vi "Get All Project VI Data.vi"(8 "error in":errorcluster, 11 "Lvproj Path":path) -> (0 "error out":errorcluster, 3 "VI Data":T1[](array[typedef]))   [LabVIEW 2020, in "VI Properties Editor.lvlib"]
doc: "Gets all VI data from a project located at <B>Path</B>."
uses:
  VI Properties Editor.lvlib
  <vilib>/xml/NI_XML.lvlib
  <vilib>/xml/Close Reference(Node).vi
  CTLs/Control Properties.ctl
  <vilib>/picture/picture.llb/imagedata.ctl
  CTLs/VI Properties.ctl
  CTLs/VI Data.ctl
  CTLs/XPath Get Attribute.ctl
  <vilib>/xml/Load XML String.vi
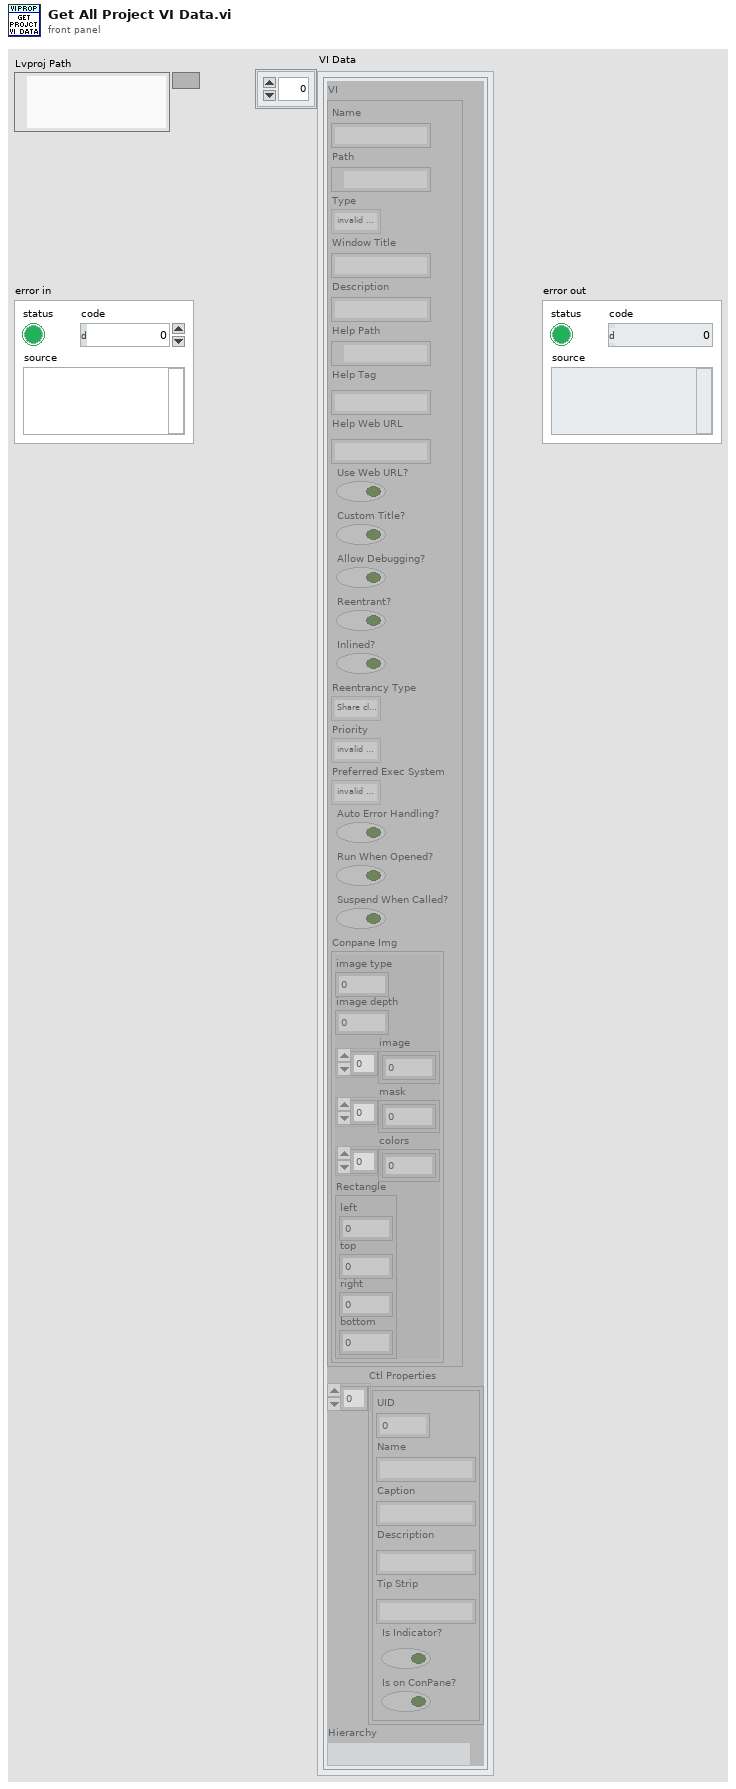
[diagram p1: front panel]
types:
  T1 = typedef "VI Properties Editor.lvlib/VI Data.ctl" = cluster{"VI":T2, "Ctl Properties":T4[], "Hierarchy":string}
  T2 = typedef "VI Properties Editor.lvlib/VI Properties.ctl" = cluster{"Name":string, "Path":path, "Type":enum32{"invalid VI type", "Standard VI", "Control VI", "Global VI", "Polymorphic VI", "Configuration VI", "SubSystem", "Facade VI", "Method VI", "Statechart Diagram VI"}, "Window Title":string, "Description":string, "Help Path":path, "Help Tag":string, "Help Web URL":string, "Use Web URL?":bool, "Custom Title?":bool, "Allow Debugging?":bool, "Reentrant?":bool, "Inlined?":bool, "Reentrancy Type":enum16{"Share clones between instances", "Preallocate clone for each instance"}, "Priority":enum32{"invalid priority", "background priority", "normal priority", "above normal priority", "high priority", "time critical priority", "subroutine"}, "Preferred Exec System":enum32{"invalid execution system", "user interface", "standard", "instrument i/o", "data acquisition", "other 1", "other 2", "same as caller"}, "Auto Error Handling?":bool, "Run When Opened?":bool, "Suspend When Called?":bool, "Conpane Img":T3}
  T3 = typedef "imagedata.ctl" = cluster{"image type":i32, "image depth":i32, "image":u8[], "mask":u8[], "colors":u32[], "Rectangle":cluster{"left":i16, "top":i16, "right":i16, "bottom":i16}}
  T4 = typedef "VI Properties Editor.lvlib/Control Properties.ctl" = cluster{"UID":i32, "Name":string, "Caption":string, "Description":string, "Tip Strip":string, "Is Indicator?":bool, "Is on ConPane?":bool}
  T5 = typedef "VI Properties Editor.lvlib/XPath Get Attribute.ctl" = enum16{"Item[@Type='VI']/@URL", "Item[@Type='LVClass']/@URL", "Item[@Type='Library']/@URL", "Item[@Type='Folder' and not (@URL)]/@Name", "@Name"}
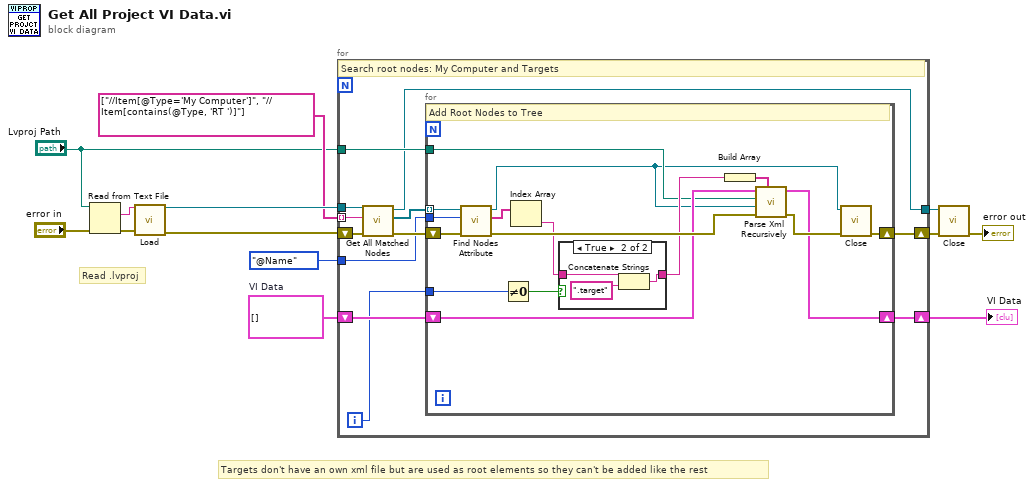
[diagram p0: block diagram]
diagram:
  w2 = T1[] []  # VI Data
  # "Targets don't have an own xml file but are used as root elements so they can't be added like the rest"
  # "Read .lvproj"
  n1 = Read from Text File(file (use dialog)="Lvproj Path", error in="error in") -> (text=w12:string, error out=w11:errorcluster)  [unwired: 2 in, 2 out]
  n2 = call-poly <vilib>:"Load.vi"("XML string"=w12, "error in (no error)"=w11) -> ("DOM document out"=w13:refnum<k20>, "error out"=w9:errorcluster)  [unwired: 11 in, 1 out]
  n3 = for {
    tunnel: w13 -> [w25]
    tunnel: string[] ["//Item[@Type='My Computer']", "//Item[contains(@Type, 'RT ')]"] -> [w24] mode=indexing
    tunnel: "Lvproj Path" -> [w23]
    shift-right: [w22] -> w10
    shift-left: w9 -> [w20]
    tunnel: [w18] -> w7
    shift-right: [w16] -> w1
    shift-left: w2 -> [w17]
    tunnel: XPath_Get_Attribute."@Name" ("XPath") -> [w15]
    i -> [w14]
    # "Search root nodes: My Computer and Targets"
    n4 = call <vilib>:"Get All Matched Nodes.vi"("error in (no error)"=w20, "XPath expression"=w24, "node in"=w25) -> ("error out"=w19:errorcluster, "node result array"=w21:refnum<k20>[], "node out"=w18:refnum<k20>)  [unwired: 6 in]
    n5 = for {
      tunnel: w23 -> [w29]
      tunnel: w21 -> [w28] mode=indexing
      shift-right: [w40] -> w22
      shift-left: w19 -> [w39]
      shift-right: [w35] -> w16
      shift-left: w17 -> [w36]
      tunnel: w15 -> [w37]
      tunnel: w14 -> [w31]
      # "Add Root Nodes to Tree"
      n6 = call "Find Nodes Attribute.vi"("error in"=w39, "XPath"=w37, "Node in"=w28) -> ("error out"=w38:errorcluster, "Attribute"=w27:string[], "Node out"=w26:refnum<k20>)  [unwired: 6 in]
      n7 = Not Equal To 0?(x=w31) -> (x != 0?=w34:bool)
      n8 = Index Array(array=w27) -> (element=w33:string)  [unwired: 1 in]
      n9 = case shown="True" w34 {
        tunnel: w33 -> [w42 w45]
        tunnel: [w42 w44] -> w32
        frame False {
        }
        frame True {
          n10 = Concatenate Strings(w45, ".target" ("string")) -> (w44:string)
        }
      }
      n11 = Build Array(w32) -> (w30:string[])
      n12 = call "Parse Xml Recursively.vi"("Parents"=w30, "error in"=w38, "DOM document in"=w26, "XML File Path"=w29, "VI Data"=w36) -> ("error out"=w41:errorcluster, "VI Data out"=w35:T1[])  [unwired: 5 in]
      n13 = call-poly <vilib>:"Close.vi"("error in (no error)"=w41, "node"=w26) -> ("error out"=w40:errorcluster)  [unwired: 7 in]
    }
  }
  "VI Data" <- w1
  n14 = call-poly <vilib>:"Close.vi"("error in (no error)"=w10, "node"=w7) -> ("error out"=→"error out":errorcluster)  [unwired: 7 in]
